vi "from string.vi"(8 "error in":errorcluster, 9 "data":string, 10 "version":string, 11 "asynchronous execution module configuration In":refnum<class "asynchronous execution module configuration.lvclass">) -> (0 "error out":errorcluster, 3 "asynchronous execution module configuration Out":refnum<class "asynchronous execution module configuration.lvclass">)   [LabVIEW 2013, in "asynchronous execution module configuration.lvclass"]
doc: "Provides an interface for loading a component configuration from a file or other serialized data source. It is recommended that all children of this class store data in two sets--data required for its own initialization, and any data required for parent initialization--and that each implementation uses the <b>Call Parent Method</b> primitive to de-serialize parent information. As a result, it is expected that every component configuration class calls <b>component configuration.lvclass:From String.vi</b>."
uses:
  asynchronous execution module configuration.lvclass
  <vilib>/NI/Tag Bus Module Framework/module configuration/TBM module configuration.lvclass
  Framework Configuration Classes/platypus configuration/class discovery singleton methods.ctl
  asynchronous execution module configuration.lvclass/asynchronous execution module configuration.ctl
  <vilib>/NI/Tag Bus Module Framework/root configuration/TBM configuration.lvclass
  Framework Configuration Classes/plugin discovery singleton/class discovery singleton.lvlib
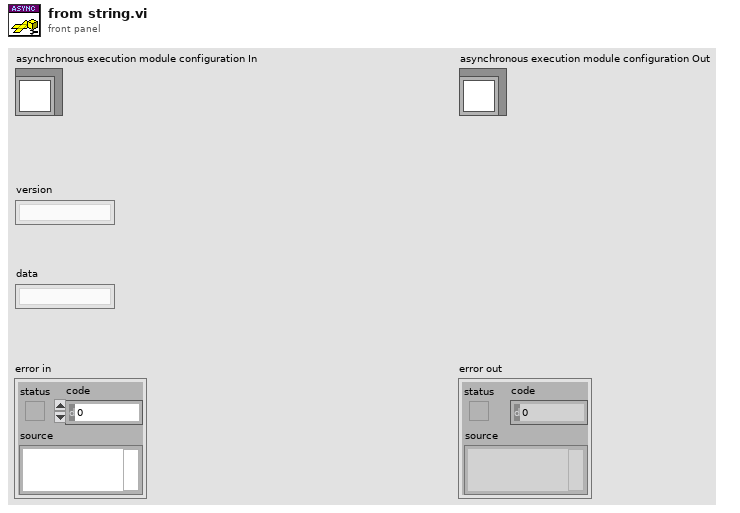
[diagram p1: front panel]
types:
  T1 = typedef "class discovery singleton.lvlib/class discovery singleton methods.ctl" = enum16{"add search paths", "load class by name", "list available classes", "get class path"}
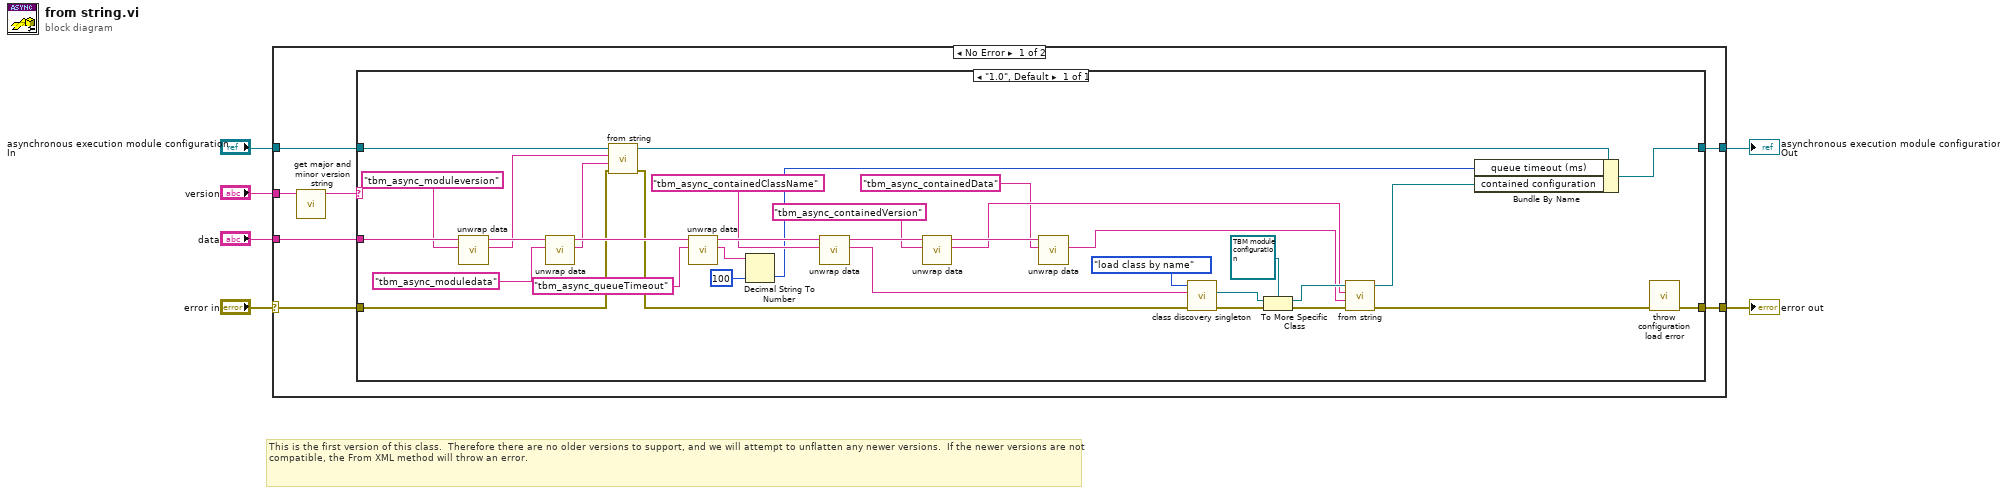
[diagram p0: block diagram]
diagram:
  # "This is the first version of this class.  Therefore there are no older versions to support, and we will attempt to unflatten any newer versions.  If the newer versions are not compatible, the From XML method will throw an error."
  n1 = case shown="No Error" "error in" {
    selector: "error in" -> [w9 w49]
    tunnel: "data" -> [w13 _]
    tunnel: "asynchronous execution module configuration In" -> [w12 w48]
    tunnel: [w11 w48] -> w5
    tunnel: [w10 w49] -> w4
    tunnel: "version" -> [w8 _]
    frame No Error {
      n2 = call <vilib>:"get major and minor version string.vi"("full version"=w8) -> ("major.minor version"=w7:string)  [unwired: 10 in]
      n3 = case shown="\"1.0\", Default" w7 {
        tunnel: w13 -> [w38]
        tunnel: w9 -> [w26]
        tunnel: w12 -> [w47]
        tunnel: [w46] -> w11
        tunnel: [w40] -> w10
        frame "1.0", Default {
          n4 = call <vilib>:"unwrap data.vi"("identifier"="tbm_async_moduleversion" ("additional identifier"), "data to unwrap"=w38) -> ("unwrapped data"=w30:string, "remaining string"=w37:string)  [unwired: 8 in]
          n5 = call <vilib>:"unwrap data.vi"("identifier"="tbm_async_moduledata" ("additional identifier"), "data to unwrap"=w37) -> ("unwrapped data"=w29:string, "remaining string"=w36:string)  [unwired: 8 in]
          n6 = call-parent "from string.vi"("error in"=w26, "data"=w29, "version"=w30, "module configuration in"=w47) -> ("error out"=w15:errorcluster, "module configuration out"=w43:refnum<class "asynchronous execution module configuration.lvclass">)  [unwired: 6 in]
          n7 = call <vilib>:"unwrap data.vi"("identifier"="tbm_async_queueTimeout" ("additional identifier"), "data to unwrap"=w36) -> ("unwrapped data"=w27:string, "remaining string"=w33:string)  [unwired: 8 in]
          n8 = Decimal String To Number(string=w27, default (0L)=100 ("queue timeout (ms)")) -> (number=w14:i32)  [unwired: 1 in, 1 out]
          n9 = call <vilib>:"unwrap data.vi"("identifier"="tbm_async_containedClassName" ("additional identifier"), "data to unwrap"=w33) -> ("unwrapped data"=w18:string, "remaining string"=w34:string)  [unwired: 8 in]
          n10 = call <vilib>:"unwrap data.vi"("identifier"="tbm_async_containedVersion" ("additional identifier"), "data to unwrap"=w34) -> ("unwrapped data"=w23:string, "remaining string"=w35:string)  [unwired: 8 in]
          n11 = call <vilib>:"unwrap data.vi"("identifier"="tbm_async_containedData" ("additional identifier"), "data to unwrap"=w35) -> ("unwrapped data"=w22:string)  [unwired: 8 in, 1 out]
          n12 = call "class discovery singleton.vi"("error in"=w15, "Class Name"=w18, "method"=class_discovery_singleton_methods."load class by name") -> ("error out"=w20:errorcluster, "LabVIEW Object"=w19:refnum<class>)  [unwired: 5 in, 2 out]
          n13 = To More Specific Class(target class=refnum<class "TBM module configuration.lvclass"> refnum ("component configuration"), reference=w19, error in=w20) -> (specific class reference=w44:refnum<class "TBM module configuration.lvclass">, error out=w45:errorcluster)
          n14 = call-dynamic "from string.vi"("error in"=w45, "data"=w22, "version"=w23, "module configuration in"=w44) -> ("error out"=w39:errorcluster, "module configuration out"=w42:refnum<class "TBM module configuration.lvclass">)  [unwired: 6 in]
          n15 = Bundle By Name(cluster=w43, "queue timeout (ms)"=w14, "contained configuration"=w42) -> (w46:refnum<class "asynchronous execution module configuration.lvclass">)
          n16 = call <vilib>:"throw configuration load error.vi"("error in"=w39) -> ("error out"=w40:errorcluster)  [unwired: 10 in]
        }
      }
    }
    frame Error {
    }
  }
  "error out" <- w4
  "asynchronous execution module configuration Out" <- w5
